vi "Read Input Samples_v1.9.vi"() -> (4 "Array":T1[](array[typedef]), 10 "output valid":bool)   [LabVIEW 2015, in "DDC_7976R_v1.lvlib"]
uses:
  DDC_7976R_v1.lvlib
  <instrlib>/_niInstr/DSP/v1/Shared/Public/IQ Data.ctl
  <vilib>/rvi/eio/common/nirviEmuTemplateMethod_errors.vi
  <vilib>/eio/EIONode/EIONode.xnode
  <instrlib>/_niInstr/DSP/v1/Shared/niInstr DSP v1 Shared.lvlib
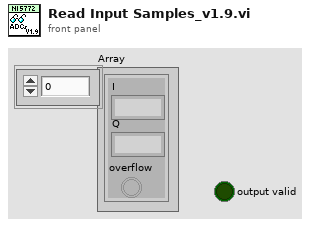
[diagram p1: front panel]
types:
  T1 = typedef "niInstr DSP v1 Shared.lvlib/IQ Data.ctl" = cluster{"I":fxp<+/-,18,1>, "Q":fxp<+/-,18,1>, "overflow":bool}
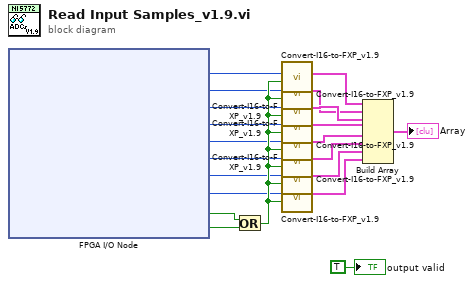
[diagram p0: block diagram]
diagram:
  n1 = xnode "FPGA I/O Node"() -> ("IO Module\\AI 1 Data N-3"=w2:i16, "IO Module\\AI 0 Data N-3"=w3:i16, "IO Module\\AI 1 Data N-2"=w4:i16, "IO Module\\AI 0 Data N-2"=w5:i16, "IO Module\\AI 1 Data N-1"=w6:i16, "IO Module\\AI 0 Data N-1"=w7:i16, "IO Module\\AI 1 Data N"=w8:i16, "IO Module\\AI 0 Data N"=w9:i16, "IO Module\\AI 0 Over Range N"=w10:bool, "IO Module\\AI 1 Over Range N"=w11:bool)  [unwired: 10 in, 10 out]
  n2 = Or(x=w10, y=w11) -> (x .or. y?=w21:bool)
  n3 = call "Convert-I16-to-FXP_v1.9.vi"("Overflow"=w21, "I16 in"=w2) -> ("data out"=w12:T1)  [unwired: 5 in]
  n4 = call "Convert-I16-to-FXP_v1.9.vi"("Overflow"=w21, "I16 in"=w3) -> ("data out"=w13:T1)  [unwired: 5 in]
  n5 = call "Convert-I16-to-FXP_v1.9.vi"("Overflow"=w21, "I16 in"=w4) -> ("data out"=w14:T1)  [unwired: 5 in]
  n6 = call "Convert-I16-to-FXP_v1.9.vi"("Overflow"=w21, "I16 in"=w5) -> ("data out"=w15:T1)  [unwired: 5 in]
  n7 = call "Convert-I16-to-FXP_v1.9.vi"("Overflow"=w21, "I16 in"=w6) -> ("data out"=w16:T1)  [unwired: 5 in]
  n8 = call "Convert-I16-to-FXP_v1.9.vi"("Overflow"=w21, "I16 in"=w7) -> ("data out"=w17:T1)  [unwired: 5 in]
  n9 = call "Convert-I16-to-FXP_v1.9.vi"("Overflow"=w21, "I16 in"=w8) -> ("data out"=w18:T1)  [unwired: 5 in]
  n10 = call "Convert-I16-to-FXP_v1.9.vi"("Overflow"=w21, "I16 in"=w9) -> ("data out"=w19:T1)  [unwired: 5 in]
  n11 = Build Array(w12, w13, w14, w15, w16, w17, w18, w19) -> (→"Array":T1[])
  "output valid" <- TRUE ("output valid")
